vi "6_STR_SubVi (1).vi"() -> ()   [LabVIEW 2020]
uses:
  Program Files (x86)/National Instruments/LabVIEW 2018/menus/Categories/IAControl Library/continuous linear.llb/Integrator (DBL).vi
  <vilib>/Analysis/NI_AALPro.lvlib
  <vilib>/Analysis/NI_AALBase.lvlib
  <vilib>/Analysis/polynomials.llb/Create Polynomial From Roots (CDB).vi
  <vilib>/Analysis/baseanly.llb/Real Dot Product.vi
  <vilib>/Analysis/Matrix/Datatypes/RealMatrix.ctl
  <vilib>/Analysis/Matrix/NI_Matrix.lvlib
panel:
  out "A":T1
  in  "stop":bool
  out "Respuesta":cluster{"TK1%":dbl, "S.P":dbl, "u(k)%":i8}(graph)
  out "Regresor(-u/e)":dbl[](array[numeric])
  out "p/q":dbl[](array[numeric]) format="%.4f"
  out "Pd(z)":dbl[](array[numeric]) format="%#_4g"
  in  "Pnd":cdb[](array[numeric])=[0.2+0.0i, 0.2+0.0i, 0.0+0.0i]
  in  "ts(s)":dbl=10.0
  in  "Tm":dbl=0.5
  in  "Mp(%)":dbl=5.0
  out "TK2 Real":dbl format="%.2f"
  out "TK1 Real":dbl format="%.2f"
  out "u(k)%":i8
  out "Theta":dbl[](array[numeric]) format="%#_4g"
  in  "Parametros":T2={"Lambda"=0.98, "Alfa"=10000.0, "nb"=2, "d"=1, "na"=2, "b0? "=FALSE}
  in  "S.P":dbl=50.0
  out "u(k) Real":dbl
  out "TK2%":dbl(slide) scale=0.0..100.0
  out "TK1%":dbl(slide) scale=0.0..100.0
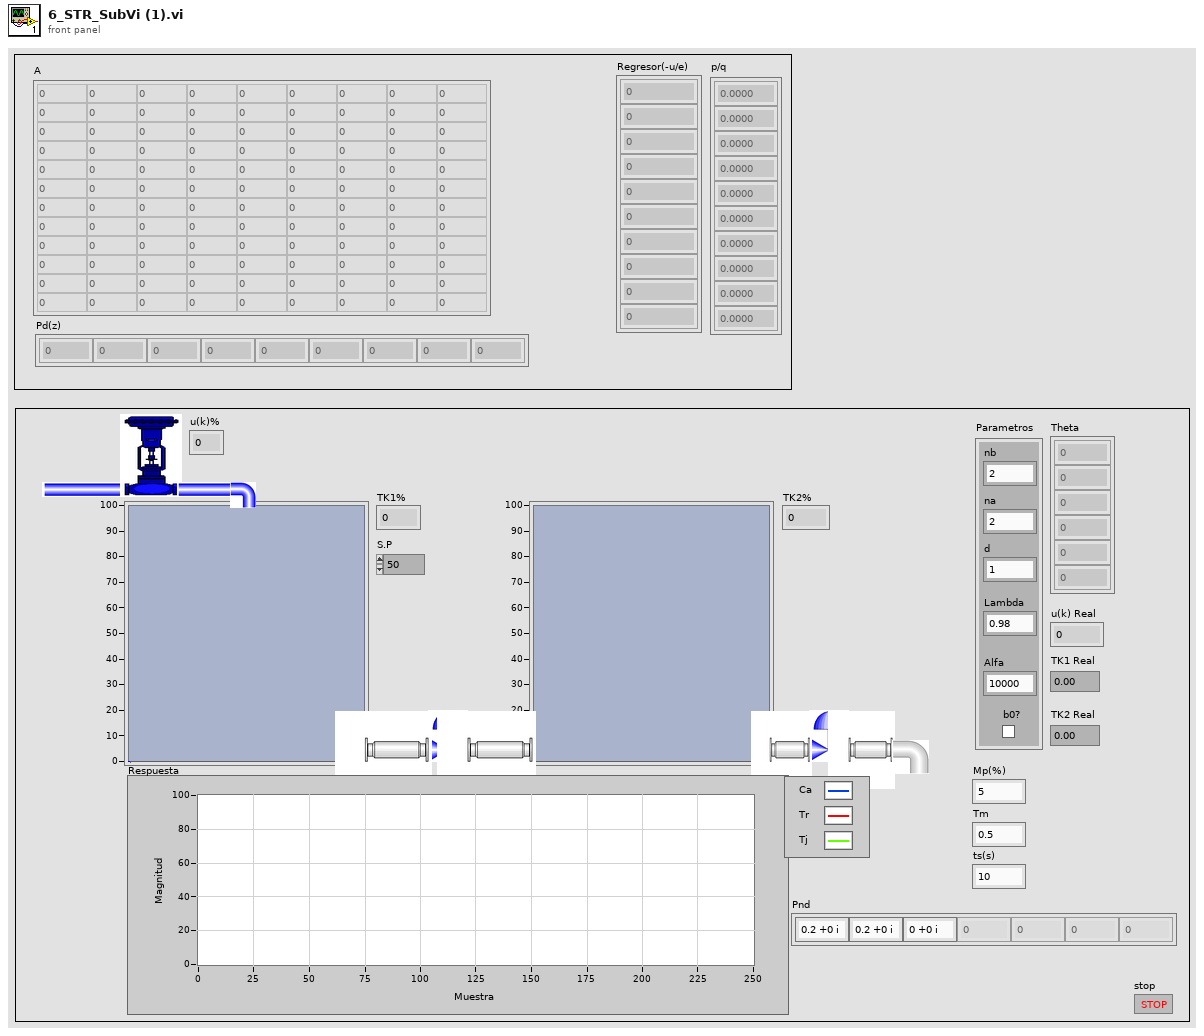
[diagram p1: front panel]
types:
  T1 = typedef "NI_Matrix.lvlib/RealMatrix.ctl" = dbl[][]
  T2 = cluster{"Lambda":dbl, "Alfa":dbl, "nb":i32, "d":i32, "na":i32, "b0? ":bool}
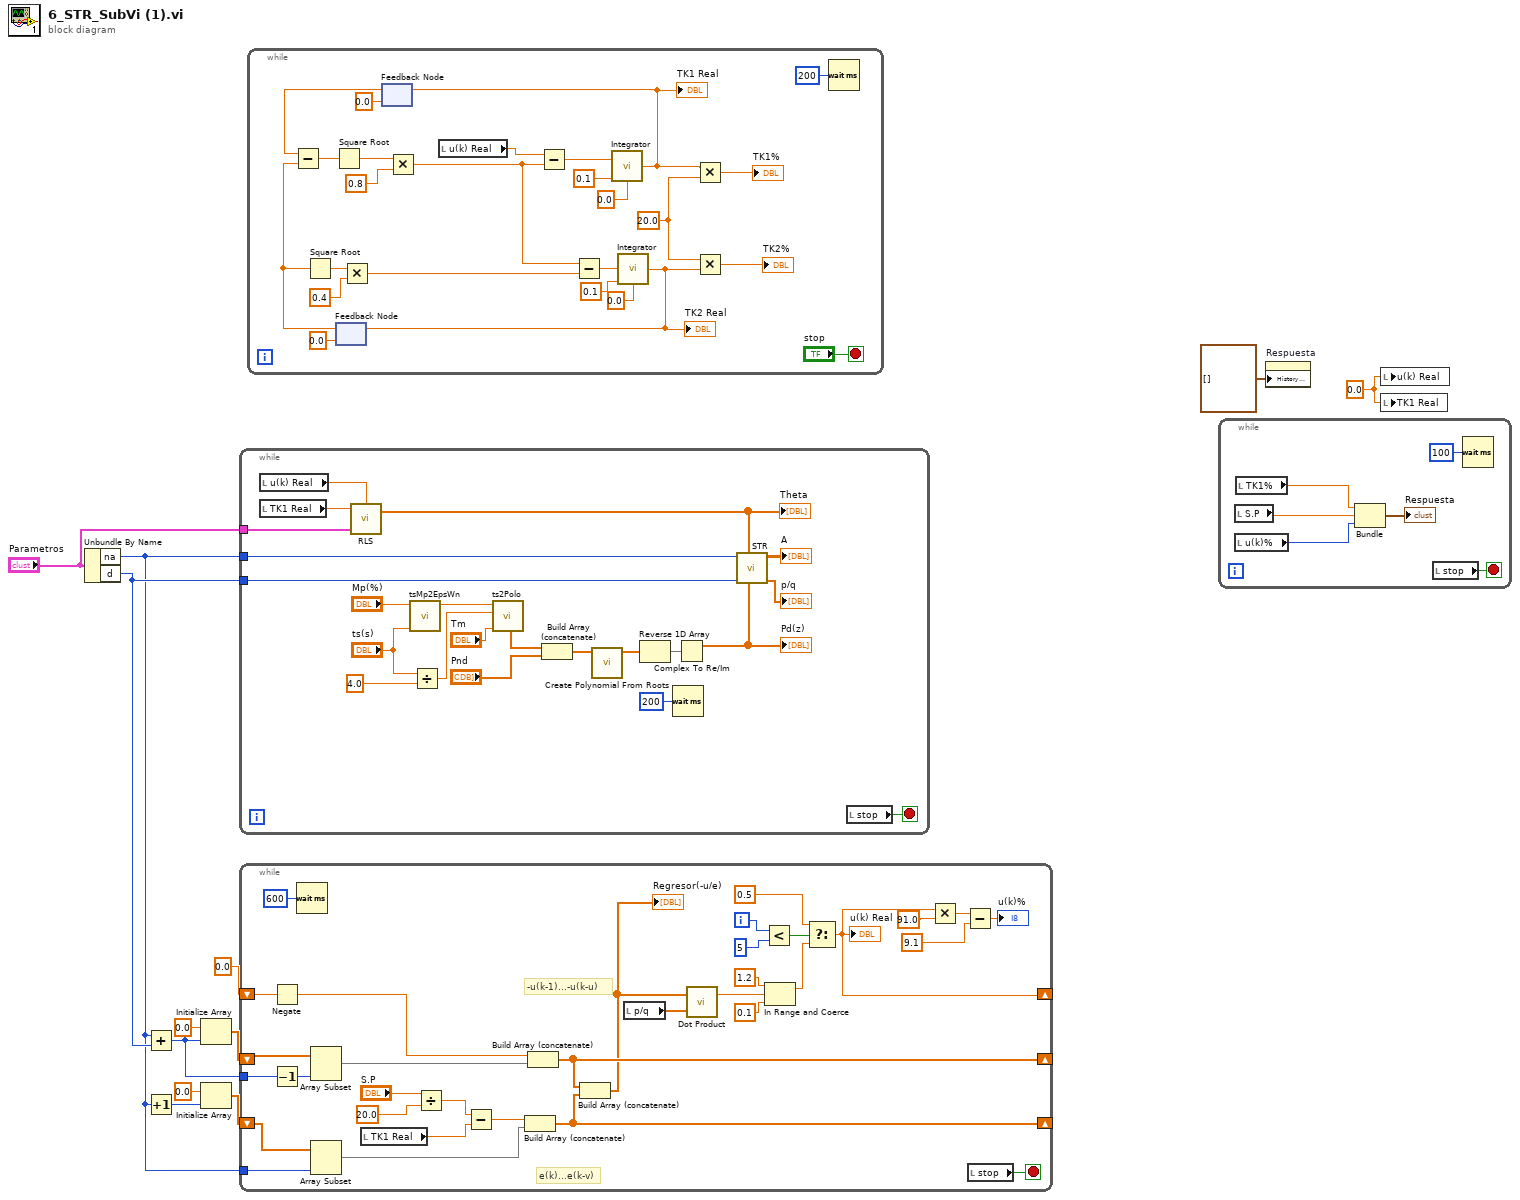
[diagram p0: block diagram]
diagram:
  w12 = 0.0 ("TK1 Real")
  n1 = Unbundle By Name("Parametros") -> ("na"=w1:i32, "d"=w2:i32)
  n2 = Add(x=w1, y=w2) -> (x+y=w5:i32)
  n3 = Increment(x=w1) -> (x+1=w9:i32)
  n4 = Initialize Array(0.0 ("element"), w5) -> (w6:dbl[])
  n5 = Initialize Array(0.0 ("element"), w9) -> (w10:dbl[])
  n6 = while {
    tunnel: "Parametros" -> [w31]
    tunnel: w1 -> [w15]
    tunnel: w2 -> [w14]
    stop <- w34 stop-if-true
    n7 = local read "u(k) Real"() -> (w29:dbl)
    n8 = local read "TK1 Real"() -> (w30:dbl)
    n9 = call "RLS.vi"("u(k)"=w29, "Parametros"=w31, "y(k)"=w30) -> ("Theta"=w18:dbl[])  [unwired: 1 in, 1 out]
    "Theta" <- w18
    n10 = call "tsMp2EpsWn.vi"("ts(s)"="ts(s)", "Mp(%)"="Mp(%)") -> ("Epsilon"=w13:dbl)  [unwired: 8 in, 1 out]
    n11 = Divide(x="ts(s)", y=4.0) -> (x/y=w25:dbl)
    n12 = call "ts2Polo.vi"("Tm"="Tm", "Tao"=w25, "Epsilon"=w13) -> ("Polos (Z1,Z2)"=w24:cdb[])  [unwired: 6 in, 2 out]
    n13 = Build Array (concatenate)(w24, "Pnd") -> (w22:cdb[])
    n14 = call-poly <vilib>:"Create Polynomial From Roots.vi"("Roots"=w22) -> ("P(x)"=w21:cdb[])  [unwired: 9 in, 1 out]
    n15 = Reverse 1D Array(array=w21) -> (reversed array=w20:cdb[])
    n16 = Wait (ms)(milliseconds to wait=u32 200) -> ()  [unwired: 1 out]
    n17 = Complex To Re/Im(x + iy=w20) -> (x=w17:dbl[])  [unwired: 1 out]
    "Pd(z)" <- w17
    n18 = call "STR.vi"("Pd(z)"=w17, "Theta in"=w18, "d"=w14, "m"=w15) -> ("p/q"=→"p/q":dbl[], "A"=→"A":T1)  [unwired: 6 in]
    n19 = local read "stop"() -> (w34:bool)
  }
  n20 = while {
    shift-right: [w56] -> _
    shift-left: w10 -> [w62]
    tunnel: w1 -> [w60]
    shift-right: [w36] -> _
    shift-left: 0.0 ("X * Y") -> [w57]
    shift-right: [w51] -> _
    shift-left: w6 -> [w55]
    tunnel: w5 -> [w52]
    i -> [w43]
    stop <- w35 stop-if-true
    # "-u(k-1)...-u(k-u)"
    # "e(k)...e(k-v)"
    n21 = Negate(x=w57) -> (-x=w50:dbl)
    n22 = Decrement(x=w52) -> (x-1=w53:i32)
    n23 = Wait (ms)(milliseconds to wait=u32 600) -> ()  [unwired: 1 out]
    n24 = Array Subset(array=w55, length=w53) -> (w54:dbl[])  [unwired: 1 in]
    n25 = Array Subset(array=w62, length=w60) -> (w61:dbl[])  [unwired: 1 in]
    n26 = local read "TK1 Real"() -> (w64:dbl)
    n27 = Divide(x="S.P", y=20.0) -> (x/y=w65:dbl)
    n28 = Subtract(x=w65, y=w64) -> (x-y=w63:dbl)
    n29 = Build Array (concatenate)(w63, w61) -> (w56:dbl[])
    n30 = Build Array (concatenate)(w50, w54) -> (w51:dbl[])
    n31 = Build Array (concatenate)(w51, w56) -> (w38:dbl[])
    "Regresor(-u/e)" <- w38
    n32 = local read "p/q"() -> (w58:dbl[])
    n33 = call-poly <vilib>:"Dot Product.vi"("Y Vector"=w58, "X Vector"=w38) -> ("X * Y"=w37:dbl)  [unwired: 1 out]
    n34 = Less?(x=w43, y=5) -> (x < y?=w41:bool)
    n35 = In Range and Coerce(upper limit=1.2, x=w37, lower limit=0.1) -> (coerced(x)=w39:dbl)  [unwired: 1 out]
    n36 = Select(t=0.5, s=w41, f=w39) -> (s? t:f=w36:dbl)
    "u(k) Real" <- w36
    n37 = Multiply(x=w36, y=91.0) -> (x*y=w49:dbl)
    n38 = Subtract(x=w49, y=9.1) -> (x-y=→"u(k)%":dbl)
    n39 = local read "stop"() -> (w35:bool)
  }
  n40 = while {
    stop <- "stop" stop-if-true
    w73 = 20.0 ("y")
    n41 = feedback #1(0.0 ("output point")) -> (w82:dbl)
    n42 = Square Root(x=w82) -> (sqrt(x)=w89:dbl)
    n43 = Multiply(x=w89, y=0.4) -> (x*y=w86:dbl)
    n44 = feedback #2(0.0 ("output point")) -> (w84:dbl)
    n45 = Subtract(x=w84, y=w82) -> (x-y=w92:dbl)
    n46 = Square Root(x=w92) -> (sqrt(x)=w91:dbl)
    n47 = Multiply(x=w91, y=0.8) -> (x*y=w87:dbl)
    n48 = local read "u(k) Real"() -> (w74:dbl)
    n49 = Subtract(x=w74, y=w87) -> (x-y=w78:dbl)
    n50 = Subtract(x=w87, y=w86) -> (x-y=w83:dbl)
    n51 = call-poly "Integrator.vi"("input point"=w78, "dt"=0.1, "initial condition"=0.0) -> ("output point"=w72:dbl)  [unwired: 12 in]
    "TK1 Real" <- w72
    n52 = feedback-in #2(w72) -> ()
    n53 = call-poly "Integrator.vi"("input point"=w83, "dt"=0.1, "initial condition"=0.0) -> ("output point"=w71:dbl)  [unwired: 12 in]
    "TK2 Real" <- w71
    n54 = feedback-in #1(w71) -> ()
    n55 = Multiply(x=w72, y=w73) -> (x*y=→"TK1%":dbl)
    n56 = Multiply(x=w73, y=w71) -> (x*y=→"TK2%":dbl)
    n57 = Wait (ms)(milliseconds to wait=u32 200) -> ()  [unwired: 1 out]
  }
  n58 = while {
    stop <- w93 stop-if-true
    n59 = local read "S.P"() -> (w95:dbl)
    n60 = local read "u(k)%"() -> (w94:i8)
    n61 = local read "TK1%"() -> (w96:dbl)
    n62 = Bundle("TK1%"=w96, "S.P"=w95, "u(k)%"=w94) -> (→"Respuesta":cluster{"TK1%":dbl, "S.P":dbl, "u(k)%":i8})  [unwired: 1 in]
    n63 = local read "stop"() -> (w93:bool)
    n64 = Wait (ms)(milliseconds to wait=u32 100) -> ()  [unwired: 1 out]
  }
  n65 = property on="Respuesta" class="WFChart (strict)"("History Data"=cluster{"TK1%":dbl, "S.P":dbl, "u(k)%":dbl}[] []) -> ()  [unwired: 2 in, 2 out]
  n66 = local write "u(k) Real"(w12) -> ()
  n67 = local write "TK1 Real"(w12) -> ()
